vi "Test_IDatabaseOpenConnection_ErrorIfCalled.vi"(8 "error in (no error)":errorcluster, 11 "TestCase in":refnum<class "Test IDatabase.lvclass">) -> (0 "error out":errorcluster, 3 "TestCase out":refnum<class "Test IDatabase.lvclass">)   [LabVIEW 2020, in "Test IDatabase.lvclass"]
uses:
  Test IDatabase.lvclass
  externals/database-interface/IDatabase/IDatabase/IDatabase.lvclass
  Test IDatabase.lvclass/Test IDatabase.ctl
  <vilib>/addons/_JKI Toolkits/VI Tester/TestCase.llb/TestCase.lvclass
  C:/Program Files/National Instruments/LabVIEW 2020/vi.lib/addons/_JKI Toolkits/VI Tester/TestCase.llb/TestCase.lvclass
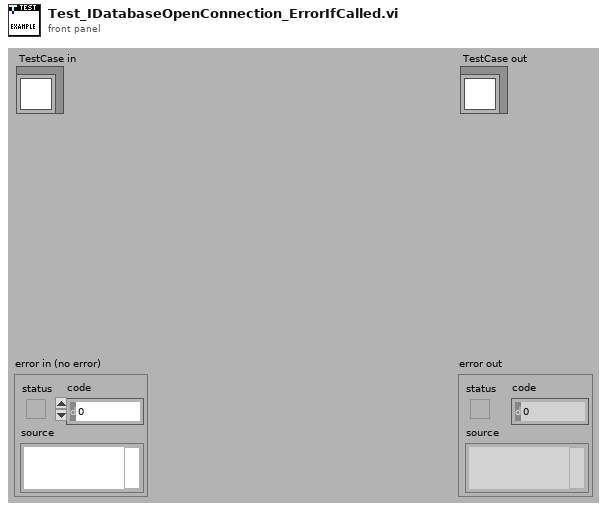
[diagram p1: front panel]
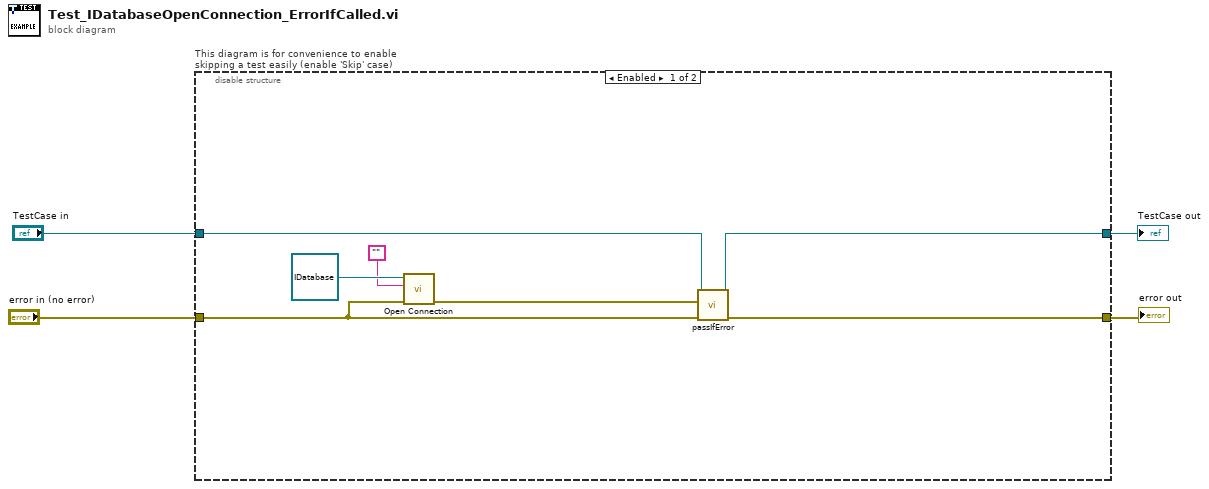
[diagram p0: block diagram]
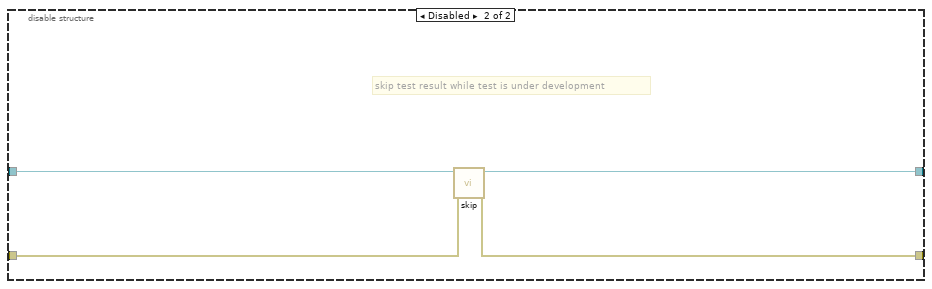
[diagram p2: hidden frame]
diagram:
  n1 = disable-structure "This diagram is for convenience to enable skipping a test easily (enable 'Skip' case)" shown="Enabled" {
    disable-tunnel: "TestCase in" -> [w11 w15]
    disable-tunnel: [w10 w13] -> w1
    disable-tunnel: [w9 w14] -> w3
    disable-tunnel: "error in (no error)" -> [w6 w12]
    frame Enabled {
      n2 = call-dynamic "Open Connection.vi"("error in (no error)"=w6, "Connection string"="", "IDatabase in"=refnum<class "IDatabase.lvclass"> refnum) -> ("error out"=w7:errorcluster)  [unwired: 7 in, 1 out]
      n3 = call-dynamic "passIfError.vi"("error in (no error)"=w6, "error"=w7, "TestCase in"=w11) -> ("error out"=w9:errorcluster, "TestCase out"=w10:refnum<class "Test IDatabase.lvclass">)  [unwired: 7 in]
    }
    frame Disabled {
      # "skip test result while test is under development"
      n4 = call <vilib>:"skip.vi"("error in (no error)"=w12, "TestCase in"=w15) -> ("error out"=w14:errorcluster, "TestCase out"=w13:refnum<class "Test IDatabase.lvclass">)  [unwired: 8 in]
    }
  }
  "error out" <- w3
  "TestCase out" <- w1
